vi "PI Build Key Array for Config.vi"(8 "error in (no error)":errorcluster, 9 "Prompted Inputs Test Parameters":T2={"Measurement"={"sxFieldId"="", "sValue"="", "nDataType"=enum."Scalar", "sUnits"="", "sDisplayName"=""}, "Limit"={"Limits On"=TRUE, "Limits"=[]}}, 10 "Template Keys (empty)":T7, 11 "Connection Refnum":T1) -> (0 "error out":errorcluster, 1 "$$INITCODE$$":string, 2 "new Template Keys":T7, 3 "Connection Refnum":T1)   [LabVIEW 2011]
uses:
  Addons/internet/utils/keyedarr.llb/Keyed Array.ctl
  TypeDefs/PI Test Parameters.ctl
  TypeDefs/PI Measurement Cluster.ctl
  TypeDefs/PI Limit Parameters.ctl
  TypeDefs/PI Limit Definition.ctl
  TypeDefs/PI Limit Comparison.ctl
  SI.LIB/ODBC/SQL Controls/Connection Refnum.ctl
  Addons/internet/utils/strutil.llb/Case Matching.ctl
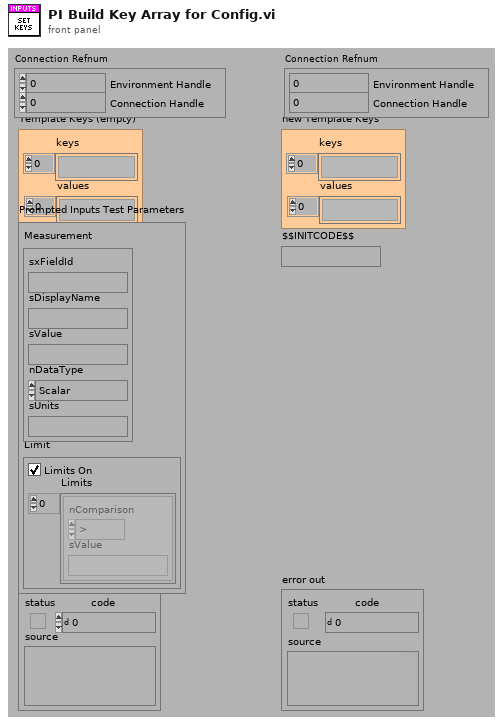
[diagram p1: front panel]
types:
  T1 = typedef "Connection Refnum.ctl" = cluster{"Environment Handle":i32, "Connection Handle":i32}
  T2 = typedef "PI Test Parameters.ctl" = cluster{"Measurement":T3, "Limit":T4}
  T3 = typedef "PI Measurement Cluster.ctl" = cluster{"sxFieldId":string, "sValue":string, "nDataType":enum16{"Scalar", "Enumeration"}, "sUnits":string, "sDisplayName":string}
  T4 = typedef "PI Limit Parameters.ctl" = cluster{"Limits On":bool, "Limits":T5[]}
  T5 = typedef "PI Limit Definition.ctl" = cluster{"nComparison":T6, "sValue":string}
  T6 = typedef "PI Limit Comparison.ctl" = enum16{">", ">=", "<", "<=", "<>", "="}
  T7 = typedef "Keyed Array.ctl" = cluster{"keys":string[], "values":string[]}
  T8 = typedef "Case Matching.ctl" = enum16{"a != A", "a == A", "system"}
  T9 = typedef "Field Record.ctl" = cluster{"ixField":i32, "iSequenceOrder":i32, "sxFieldId":string, "sxSequenceId":string, "sDisplayName":string, "sValue":string, "sUnits":string, "nDataType":T10, "nNextItem":T11, "fSystem":bool, "fSystemValue":bool, "fRequired":bool, "fSetAtTest":bool, "fTestField":bool, "fDeleted":bool, "fIndexed":bool, "fFreeList":bool}
  T10 = typedef "Field DataTypes.ctl" = enum32{"text", "numeric", "list", "timestamp", "boolean"}
  T11 = typedef "Field NextItem.ctl" = enum32{"Reset", "Retain", "Auto-Increment"}
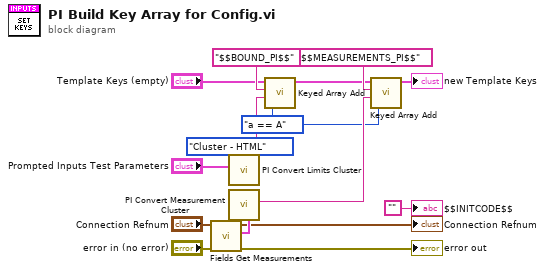
[diagram p0: block diagram]
diagram:
  w6 = Case_Matching."a == A" ("case matching (sensitive)")
  n1 = call "Fields Get Measurements.vi"("error in (no error)"="error in (no error)", "Connection Refnum"="Connection Refnum") -> ("error out"=→"error out":errorcluster, "Measurement Fields"=w12:T9[], "dup Connection Refnum"=→"Connection Refnum":T1)  [unwired: 1 in, 6 out]
  n2 = call "PI Convert Limits Cluster.vi"("Conversion"=enum16{"Cluster - HTML", "HTML - Cluster"}."Cluster - HTML", "PI Cluster In"="Prompted Inputs Test Parameters") -> ("PI HTML Out"=w13:string)  [unwired: 2 in, 5 out]
  n3 = call "PI Convert Measurement Cluster.vi"("PI Measurement Field Array"=w12) -> ("PI HTML Out"=w8:string)  [unwired: 1 in, 7 out]
  n4 = call "Keyed Array Add.vi"("case matching (sensitive)"=w6, "value"=w13, "key"="$$BOUND_PI$$", "array in"="Template Keys (empty)") -> ("array out"=w10:T7)  [unwired: 3 out]
  n5 = call "Keyed Array Add.vi"("case matching (sensitive)"=w6, "value"=w8, "key"="$$MEASUREMENTS_PI$$", "array in"=w10) -> ("array out"=→"new Template Keys":T7)  [unwired: 3 out]
  "$$INITCODE$$" <- ""
